vi "Drive Controller.vi"(8 "error in":errorcluster) -> ()   [LabVIEW 2015]
doc: "This VI executes continuously carrying out the current operation and responding to updates or new operation requests. It will often contain the timing or control code that is difficult to place directly in TeleOp. This VI generally opens all sensors and motors and isolates the rest of the robot code from knowing implementation details of how the operations are carried out."
uses:
  <vilib>/Rock Robotics/WPI/CAN/TalonSRX/WPI_CANTalonSRX_GlobalStatus.ctl
  Drive Setpoints.ctl
  Drive Operations.ctl
  <vilib>/Rock Robotics/WPI/SafetyOutput/WPI_SafetyOutputConfigMenu.ctl
  <vilib>/Rock Robotics/WPI/CAN/TalonSRX/WPI_CANTalonSRX_APIControlMode.ctl
  JoystickData.ctl
  <vilib>/Rock Robotics/WPI/MotorControl/WPI_MotorControlOpenCANTalonSRX.vi
  <vilib>/Rock Robotics/WPI/Utilities/WPI_GetSetVariantRefNum.vi
  Global Drive Variables.vi
  LED Lights/LED Lights Global.vi
panel:
  out "Talon SRX Status 2":T1
  out "Talon SRX Status":T1
  out "Setpoints":T2(graph)
  out "Current\nCmd":string
  # "Tip: It may be helpful to observe inputs and sensor values.\nYou may also want to display tuning or debugging controls."
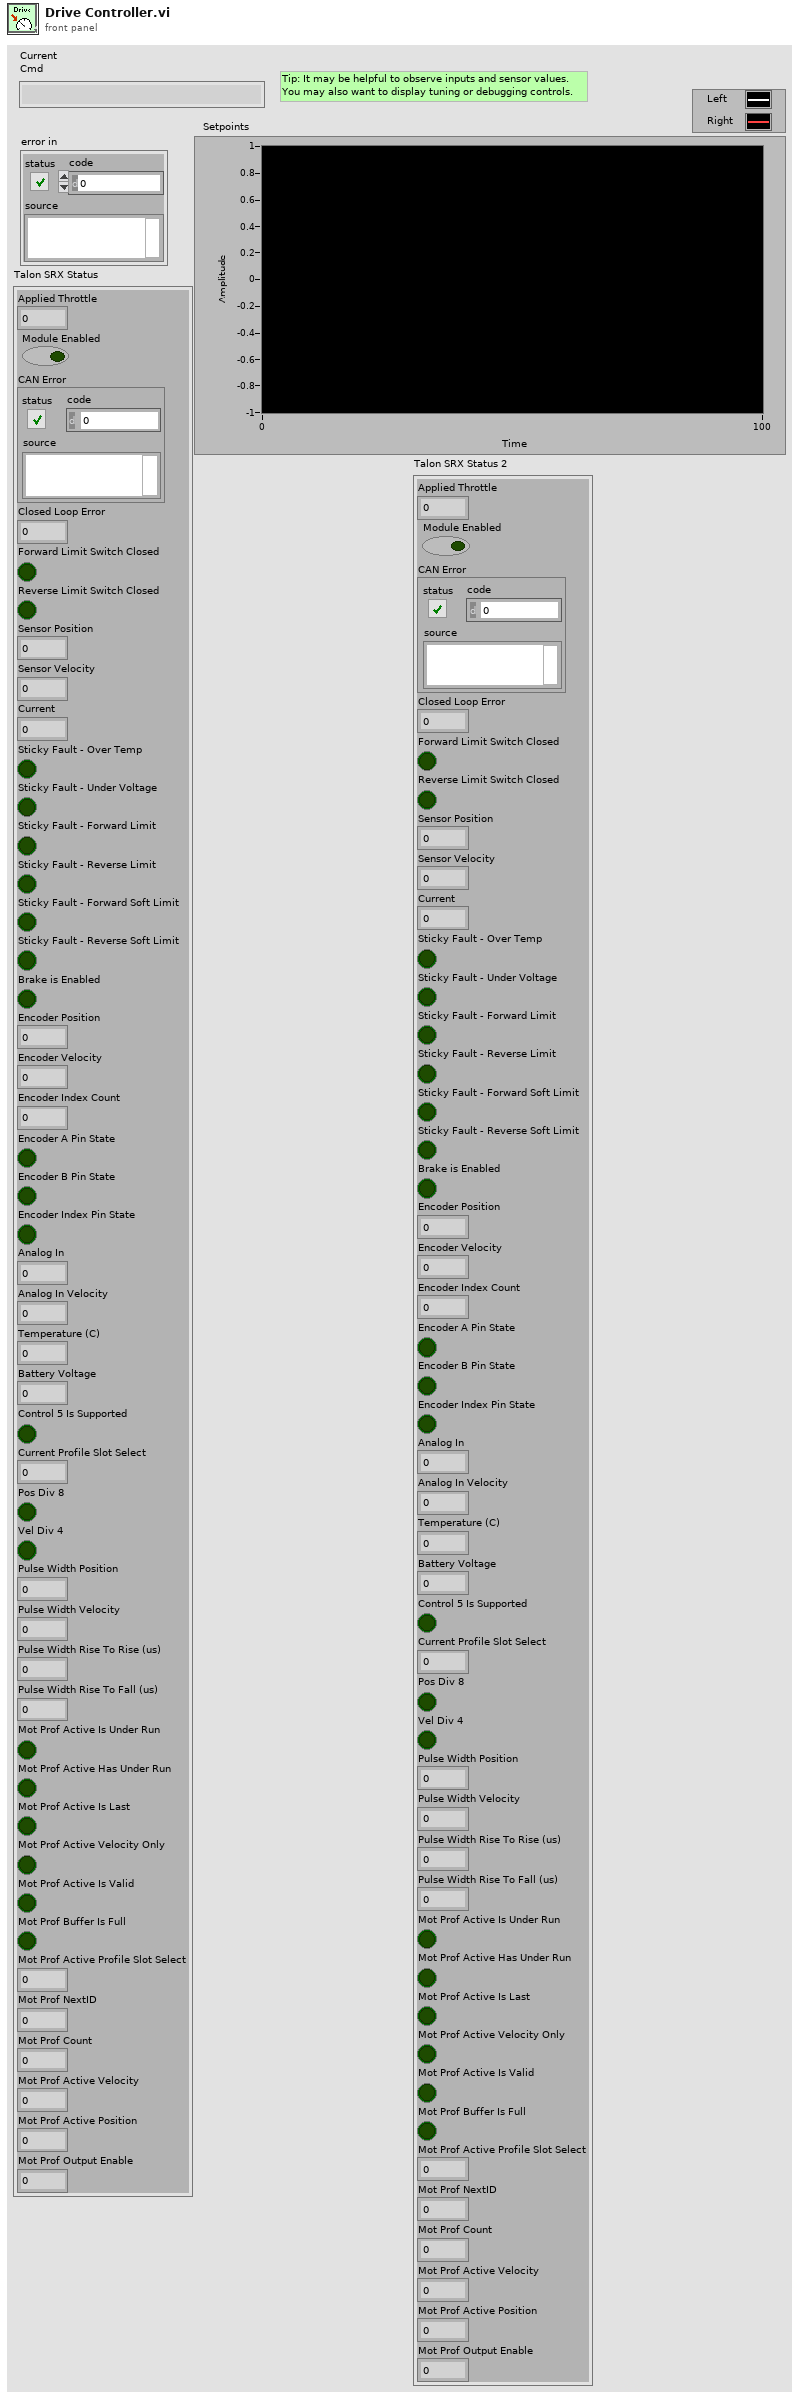
[diagram p1: front panel]
types:
  T1 = typedef "WPI_CANTalonSRX_GlobalStatus.ctl" = cluster{"Applied Throttle":dbl, "Module Enabled":bool, "CAN Error":errorcluster, "Closed Loop Error":dbl, "Forward Limit Switch Closed":bool, "Reverse Limit Switch Closed":bool, "Sensor Position":dbl, "Sensor Velocity":dbl, "Current":dbl, "Sticky Fault - Over Temp":bool, "Sticky Fault - Under Voltage":bool, "Sticky Fault - Forward Limit":bool, "Sticky Fault - Reverse Limit":bool, "Sticky Fault - Forward Soft Limit":bool, "Sticky Fault - Reverse Soft Limit":bool, "Brake is Enabled":bool, "Encoder Position":dbl, "Encoder Velocity":dbl, "Encoder Index Count":dbl, "Encoder A Pin State":bool, "Encoder B Pin State":bool, "Encoder Index Pin State":bool, "Analog In":dbl, "Analog In Velocity":dbl, "Temperature (C)":dbl, "Battery Voltage":dbl, "Control 5 Is Supported":bool, "Current Profile Slot Select":dbl, "Pos Div 8":bool, "Vel Div 4":bool, "Pulse Width Position":i32, "Pulse Width Velocity":i32, "Pulse Width Rise To Rise (us)":i32, "Pulse Width Rise To Fall (us)":i32, "Mot Prof Active Is Under Run":bool, "Mot Prof Active Has Under Run":bool, "Mot Prof Active Is Last":bool, "Mot Prof Active Velocity Only":bool, "Mot Prof Active Is Valid":bool, "Mot Prof Buffer Is Full":bool, "Mot Prof Active Profile Slot Select":i32, "Mot Prof NextID":i32, "Mot Prof Count":i32, "Mot Prof Active Velocity":dbl, "Mot Prof Active Position":dbl, "Mot Prof Output Enable":i32}
  T2 = cluster{"Left Setpoint":dbl, "Right Setpoint":dbl}
  T3 = typedef "WPI_CANTalonSRX_APIControlMode.ctl" = enum8{"Percent VBus", "Speed", "Position", "Slave", "Unchanged / Invalid", "Voltage Compensation", "Current", "Motion Profile"}
  T4 = typedef "WPI_SafetyOutputConfigMenu.ctl" = enum16{"Enable", "Disable"}
  T5 = typedef "Drive Setpoints.ctl" = cluster{"Operation":T6, "Left Setpoint":dbl, "Right Setpoint":dbl, "Duration":dbl}
  T6 = typedef "Drive Operations.ctl" = enum16{"Reserve", "Read Current", "Immediate", "Drive for Time", "Drive for Distance"}
  T7 = typedef "Drive Global Type Def.ctl" = cluster{"Left Drive Motors":cluster{"Motor Front":T8, "Motor Back":T8, "Motor Errors":errorcluster}, "Right Drive Motors":cluster{"Motor Front":T8, "Motor Back":T8, "Motor Errors":errorcluster}}
  T8 = typedef "Motor Global Type Def.ctl" = cluster{"Motor Error":errorcluster}
  T9 = typedef "WPI_MotorControlDeviceRef.ctl" = cluster{"DeviceStatus":errorcluster, "Type":T10, "PWM":cluster{"PWM Channel":T11, "DeadBand":T12}, "CAN":cluster{"Device Number":u8, "Control Mode":T13, "Semaphore":T14, "Max Vout":dbl, "TalonSRX Control Mode":T3}, "Invert":bool}
  T10 = typedef "WPI_MotorControlType.ctl" = enum16{"PWM", "CAN", "CANTalonSRX"}
  T11 = typedef "FPGA_DIOPWMChannel.ctl" = enum8{"PWM 0", "PWM 1", "PWM 2", "PWM 3", "PWM 4", "PWM 5", "PWM 6", "PWM 7", "PWM 8", "PWM 9", "PWM MXP 0", "PWM MXP 1", "PWM MXP 2", "PWM MXP 3", "PWM MXP 4", "PWM MXP 5", "PWM MXP 6", "PWM MXP 7", "PWM MXP 8", "PWM MXP 9", "Invalid"}
  T12 = typedef "WPI_PWMDeadband.ctl" = cluster{"Name":string, "maxPositivePwm":i32, "minPositivePwm":i32, "centerPwm":i32, "maxNegativePwm":i32, "minNegativePwm":i32, "angularRange":u16}
  T13 = typedef "WPI_CANJaguar_ControlMode.ctl" = enum8{"Percent VBus", "Current", "Speed", "Position", "Voltage"}
  T14 = typedef "Semaphore RefNum" = refnum<k1>
  T15 = typedef "WPI_RobotDriveDevRef.ctl" = cluster{"DevStatus":errorcluster, "Motors[]":T9[], "Square Inputs":bool, "Max Output":dbl}
  T16 = typedef "Command Status Info.ctl" = cluster{"Name":string, "Status":T17, "notifier out":T18}
  T17 = typedef "Completion Status.ctl" = enum16{"Successful", "Aborted", "Incomplete"}
  T18 = typedef "Completion Notifier.ctl" = refnum<notifier>
  T19 = cluster{"SubSystem Data":T5, cluster{"Start Time (ms)":u32, "Iterations":i32}, cluster{"Command Info":T16, "Description":string, "SubSystem Data":T5, "notifier out":refnum<notifier>, "Subsystem Name":string}}
  T20 = cluster{"SubSystem Data":T5, cluster{"Start Time (ms)":u32, "Iterations":i32}, "Default Command Arguments":cluster{"Command Info":T16, "Description":string, "SubSystem Data":T5, "notifier out":refnum<notifier>, "Subsystem Name":string}}
  T21 = cluster{"Don't move motors while reserved":dbl, "Don't move motors while reserved":dbl}
  T22 = typedef "JoystickData.ctl" = cluster{"Axes":dbl[], "Buttons":bool[]}
  T23 = typedef "WPI_JoystickDevRef.ctl" = cluster{"Device":T24}
  T24 = typedef "WPI_JoystickDeviceEnum.ctl" = enum16{"USB 0", "USB 1", "USB 2", "USB 3", "USB 4", "USB 5"}
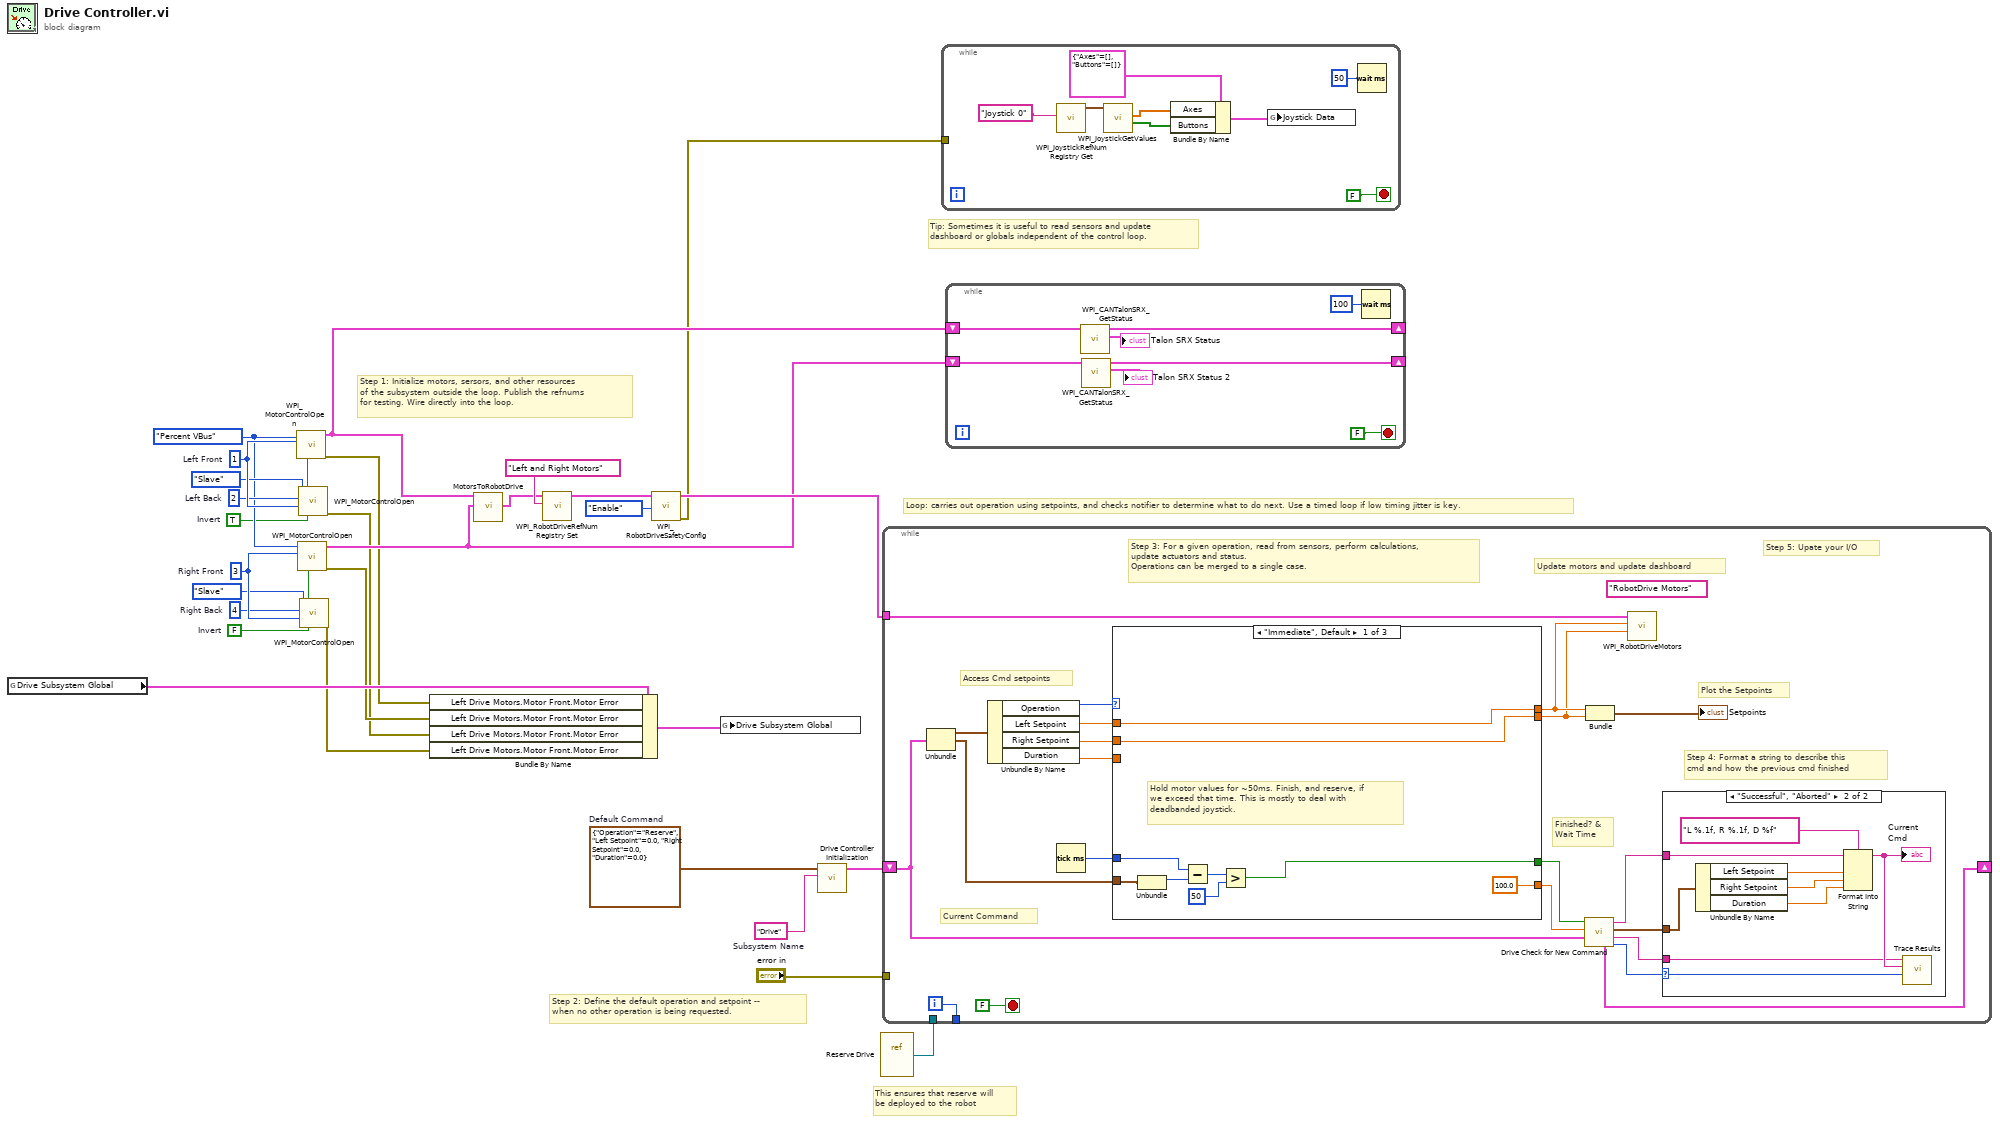
[diagram p0: block diagram]
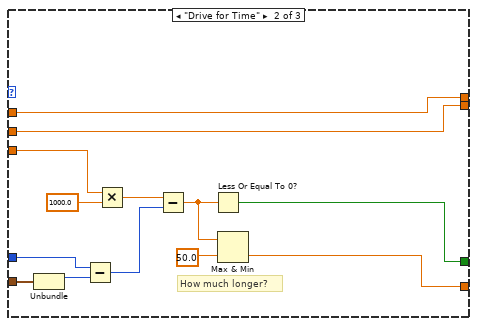
[diagram p3: hidden frame]
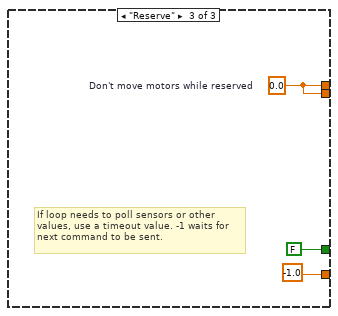
[diagram p4: hidden frame]
diagram:
  w8 = TRUE  # Invert
  w9 = FALSE  # Invert
  w14 = u8 4  # Right Back
  w15 = u8 3  # Right Front
  w17 = u8 2  # Left Back
  w18 = u8 1  # Left Front
  w12 = WPI_CANTalonSRX_APIControlMode."Percent VBus" ("Control Mode")
  w27 = T5 {"Operation"=enum."Reserve", "Left Setpoint"=0.0, "Right Setpoint"=0.0, "Duration"=0.0}  # Default Command
  w28 = "Drive"  # Subsystem Name
  # "This ensures that reserve will\nbe deployed to the robot"
  # "Tip: Sometimes it is useful to read sensors and update\ndashboard or globals independent of the control loop."
  # "Step 2: Define the default operation and setpoint --\nwhen no other operation is being requested."
  # "Step 1: Initialize motors, sersors, and other resources\nof the subsystem outside the loop. Publish the refnums\nfor testing. Wire directly into the loop."
  # "Loop: carries out operation using setpoints, and checks notifier to determine what to do next. Use a timed loop if low timing jitter is key."
  n1 = global read "LED Lights Global.vi" "Drive Subsystem Global"() -> (w6:T7)
  n2 = call-poly <vilib>:"WPI_MotorControlOpen.vi"("Invert"=w8, "Device Number"=w18, "Control Mode"=w12) -> ("error out"=w5:errorcluster, "MotorControlDeviceRef"=w11:T9)  [unwired: 7 in]
  n3 = call-poly <vilib>:"WPI_MotorControlOpen.vi"("Invert"=w9, "Device Number"=w15, "Control Mode"=w12) -> ("error out"=w4:errorcluster, "MotorControlDeviceRef"=w10:T9)  [unwired: 7 in]
  n4 = call-poly <vilib>:"WPI_MotorControlOpen.vi"("Master Device Number"=w18, "Device Number"=w17, "Control Mode"=WPI_CANTalonSRX_APIControlMode."Slave") -> ("error out"=w3:errorcluster)  [unwired: 7 in, 1 out]
  n5 = call-poly <vilib>:"WPI_MotorControlOpen.vi"("Master Device Number"=w15, "Device Number"=w14, "Control Mode"=WPI_CANTalonSRX_APIControlMode."Slave") -> ("error out"=w2:errorcluster)  [unwired: 7 in, 1 out]
  n6 = Bundle By Name(cluster=w6, "Left Drive Motors.Motor Front.Motor Error"=w5, "Left Drive Motors.Motor Front.Motor Error"=w4, "Left Drive Motors.Motor Front.Motor Error"=w3, "Left Drive Motors.Motor Front.Motor Error"=w2) -> (w1:T7)
  n7 = call "MotorsToRobotDrive.vi"("Left"=w11, "Right"=w10) -> ("RobotDriveDevRef"=w19:T15)  [unwired: 16 in, 1 out]
  n8 = call <vilib>:"WPI_RobotDriveRefNum Registry Set.vi"("refnum name"="Left and Right Motors", "RobotDriveDevRef"=w19) -> ("RobotDriveDevRef"=w25:T15)  [unwired: 2 in, 7 out]
  n9 = call <vilib>:"WPI_RobotDriveSafetyConfig.vi"("mode"=WPI_SafetyOutputConfigMenu."Enable", "RobotDriveDevRef"=w25) -> ("error out"=w7:errorcluster, "RobotDriveDevRef"=w23:T15)  [unwired: 8 in]
  n10 = global write "LED Lights Global.vi" "Drive Subsystem Global"(w1) -> ()
  n11 = call "Drive Controller Initialization.vi"("Subsystem Name"=w28, "Default Command"=w27) -> ("output cluster"=w21:T19)  [unwired: 9 in]
  n12 = vi-ref "Reserve Drive.vi"() -> (w20:refnum<vi>)
  n13 = while {
    shift-right: [w36] -> _
    shift-left: w21 -> [w29]
    tunnel: [w48] -> _
    tunnel: w23 -> [w44]
    tunnel: "error in" -> [_]
    tunnel: w20 -> [_]
    i -> [w48]
    stop <- FALSE stop-if-true
    (unwired) "RobotDrive Motors" ("Name")
    # "Step 5: Upate your I/O"
    # "Step 4: Format a string to describe this\ncmd and how the previous cmd finished"
    # "Current Command"
    # "Update motors and update dashboard"
    # "Plot the Setpoints"
    # "Access Cmd setpoints"
    # "Finished? &\nWait Time"
    # "Step 3: For a given operation, read from sensors, perform calculations,\nupdate actuators and status.\nOperations can be merged to a single case."
    n14 = Unbundle(w29) -> ("SubSystem Data"=w43:T5, w30:cluster{"Start Time (ms)":u32, "Iterations":i32})  [unwired: 1 out]
    n15 = Unbundle By Name(w43) -> ("Operation"=w42:T6, "Left Setpoint"=w41:dbl, "Right Setpoint"=w40:dbl, "Duration"=w39:dbl)
    n16 = Tick Count (ms)() -> (millisecond timer value=w38:u32)
    n17 = case shown="\"Immediate\", Default" w42 {
      tunnel: [100.0 w68 -1.0] -> w35
      tunnel: [w60 w75 FALSE ("ignore previous (F)")] -> w34
      tunnel: w30 -> [w59 w77 _]
      tunnel: [w66 w74 w81] -> w46
      tunnel: [w65 w73 w81] -> w45
      tunnel: w41 -> [w66 w74 _]
      tunnel: w40 -> [w65 w73 _]
      tunnel: w39 -> [_ w72 _]
      tunnel: w38 -> [w61 w71 _]
      frame "Immediate", Default {
        # "Hold motor values for ~50ms. Finish, and reserve, if\nwe exceed that time. This is mostly to deal with\ndeadbanded joystick."
        n18 = Unbundle(w59) -> ("Start Time (ms)"=w62:u32)  [unwired: 1 out]
        n19 = Subtract(x=w61, y=w62) -> (x-y=w63:u32)
        n20 = Greater?(x=w63, y=u8 50 ("Left Motor")) -> (0:w60:bool)
      }
      frame "Drive for Time" {
        # "How much longer?"
        n21 = Unbundle(w77) -> ("Start Time (ms)"=w76:u32)  [unwired: 1 out]
        n22 = Subtract(x=w71, y=w76) -> (x-y=w80:u32)
        n23 = Multiply(x=w72, y=1000.0) -> (x*y=w79:dbl)
        n24 = Subtract(x=w79, y=w80) -> (x-y=w70:dbl)
        n25 = Less Or Equal To 0?(x=w70) -> (x <= 0?=w75:bool)
        n26 = Max & Min(x=w70, y=50.0) -> (min(x,y)=w68:dbl)  [unwired: 1 out]
      }
      frame "Reserve" {
        w81 = 0.0  # Don't move motors while reserved
        # "If loop needs to poll sensors or other\nvalues, use a timeout value. -1 waits for\nnext command to be sent."
      }
    }
    n27 = call "Drive Check for New Command.vi"("input cluster"=w29, "Wait time (ms)"=w35, "Finished?"=w34) -> ("Completion"=w37:T17, "Subsystem Name"=w31:string, "SetPoint"=w32:T5, "Initial Trace String"=w33:string, "output cluster"=w36:T20)  [unwired: 4 in]
    n28 = Bundle("Don't move motors while reserved"=w46, "Don't move motors while reserved"=w45) -> (→"Setpoints":T21)  [unwired: 1 in]
    n29 = call <vilib>:"WPI_RobotDriveMotors.vi"("RightSpeed"=w45, "LeftSpeed"=w46, "RobotDriveDevRef"=w44) -> ()  [unwired: 1 in, 8 out]
    n30 = case shown="\"Successful\", \"Aborted\"" w37 {
      selector: w37 -> [_ w58]
      tunnel: w33 -> [_ w53]
      tunnel: w32 -> [_ w54]
      tunnel: w31 -> [_ w50]
      frame "Incomplete", Default {
        # "Continuing current command"
      }
      frame "Successful", "Aborted" {
        # "Report and setup for next command"
        n31 = Unbundle By Name(w54) -> ("Left Setpoint"=w56:dbl, "Right Setpoint"=w57:dbl, "Duration"=w51:dbl)
        n32 = Format Into String(format string="L %.1f, R %.1f, D %f", initial string=w53, w56, w57, w51) -> (resulting string=w52:string)  [unwired: 1 in, 1 out]
        "Current\nCmd" <- w52
        n33 = call <vilib>:"Trace Results.vi"("Status of previous command"=w58, "Description"=w52, "Subsystem"=w50) -> ()  [unwired: 9 in]
      }
    }
  }
  n34 = while {
    tunnel: w7 -> [_]
    stop <- FALSE stop-if-true
    n35 = call <vilib>:"WPI_JoystickRefNum Registry Get.vi"("refnum name"="Joystick 0") -> ("JoystickDevRef"=w89:T23)  [unwired: 1 in, 9 out]
    n36 = call <vilib>:"WPI_JoystickGetValues.vi"("JoystickDevRef"=w89) -> ("Buttons"=w85:bool[], "Axes"=w86:dbl[])  [unwired: 6 in, 3 out]
    n37 = Bundle By Name(cluster=T22 {"Axes"=[], "Buttons"=[]} ("Joystick Data"), "Axes"=w86, "Buttons"=w85) -> (w84:T22)
    n38 = global write "Global Drive Variables.vi" "Joystick Data"(w84) -> ()
    n39 = Wait (ms)(milliseconds to wait=u32 50) -> ()  [unwired: 1 out]
  }
  n40 = while {
    shift-right: [w96] -> _
    shift-left: w11 -> [w97]
    shift-right: [w93] -> _
    shift-left: w10 -> [w94]
    stop <- FALSE stop-if-true
    n41 = call <vilib>:"WPI_CANTalonSRX_GetStatus.vi"("CAN Talon SRX Ref"=w97) -> ("Talon SRX Status"=→"Talon SRX Status":T1, "CAN Talon SRX Ref"=w96:T9)  [unwired: 8 in, 1 out]
    n42 = call <vilib>:"WPI_CANTalonSRX_GetStatus.vi"("CAN Talon SRX Ref"=w94) -> ("Talon SRX Status"=→"Talon SRX Status 2":T1, "CAN Talon SRX Ref"=w93:T9)  [unwired: 8 in, 1 out]
    n43 = Wait (ms)(milliseconds to wait=u32 100) -> ()  [unwired: 1 out]
  }
